vi "Get All.vi"(8 "error in (no error)":errorcluster, 11 "Store in":refnum<class "Store.lvclass">) -> (0 "error out":errorcluster, 1 "Values":variant[](array[variant]), 2 "Keys":variant[](array[variant]), 3 "Store out":refnum<class "Store.lvclass">)   [LabVIEW 2018, in "Application.lvlib" / "Store.lvclass"]
uses:
  Store.lvclass
  Store.lvclass/Store.ctl
  Controls/Packet.ctl
  Dictionary Class/Dictionary.lvclass/Dictionary.ctl
  1b7bc760-b481-47a7-9710-96281ada8069.vi
  Dictionary Class/VIs/Get Data DVR.vi
  Dictionary Class/Dictionary.lvclass
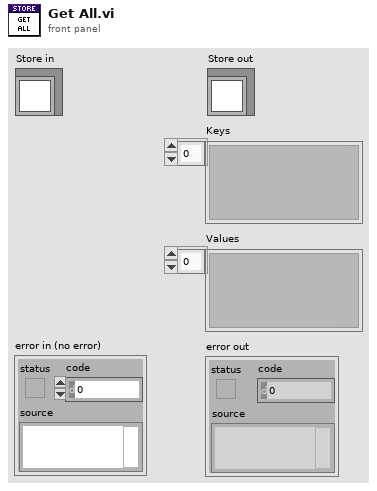
[diagram p1: front panel]
types:
  T1 = typedef "Application.lvlib/Store.lvclass/Packet.ctl" = cluster{"Type Descriptor":i16[], "Value":variant}
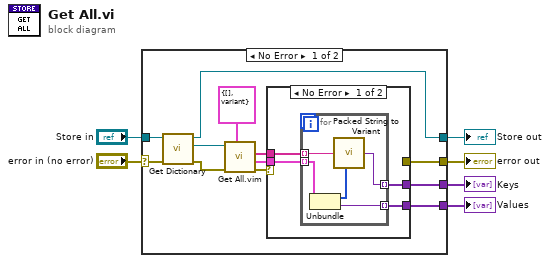
[diagram p0: block diagram]
diagram:
  n1 = case shown="No Error" "error in (no error)" {
    selector: "error in (no error)" -> [w17 w30]
    tunnel: [w8 w30] -> w5
    tunnel: [w7 w29] -> w3
    tunnel: "Store in" -> [w18 w29]
    tunnel: [w11 _] -> w2
    tunnel: [w10 _] -> w1
    frame No Error {
      n2 = call "Get Dictionary.vi"("error in (no error)"=w17, "Store in"=w18) -> ("error out"=w16:errorcluster, "Dictionary.lvclass"=w15:refnum<class "Dictionary.lvclass">, "Store out"=w7:refnum<class "Store.lvclass">)  [unwired: 7 in]
      n3 = call "Get All.vim"("Base Type"=T1 {"Type Descriptor"=[], "Value"=variant} ("Packet"), "error in (no error)"=w16, "Dictionary in"=w15) -> ("error out"=w9:errorcluster, "Values"=w12:T1[], "Names"=w13:string[])  [unwired: 5 in, 1 out]
      n4 = case shown="No Error" w9 {
        selector: w9 -> [_ w28]
        tunnel: w13 -> [w22 _]
        tunnel: w12 -> [w21 _]
        tunnel: [w20 _] -> w11
        tunnel: [w19 _] -> w10
        tunnel: [_ w28] -> w8
        frame No Error {
          n5 = for {
            tunnel: w22 -> [w25] mode=indexing
            tunnel: w21 -> [w27] mode=indexing
            tunnel: [w26] -> w20 mode=indexing
            tunnel: [w23] -> w19 mode=indexing
            n6 = Unbundle(w27) -> ("Type Descriptor"=w24:i16[], "Value"=w26:variant)
            n7 = call "Packed String to Variant.vi"("Packed String"=w25, "Type Descriptor"=w24) -> ("Variant"=w23:variant)  [unwired: 3 in]
          }
        }
        frame Error {
        }
      }
    }
    frame Error {
    }
  }
  "error out" <- w5
  "Store out" <- w3
  "Values" <- w2
  "Keys" <- w1
